vi "Teleop.vi"(10 "Match Info":T1={"Autonomous Elapsed Seconds"=0.0, "TeleOp Elapsed Seconds"=0.0, "Disabled Elapsed Seconds"=0.0, "Visited Autonomous"=FALSE, "Visited TeleOp"=FALSE, "Visited Disabled"=FALSE, "Autonomous Settings"={"Autonomous Style"=enum."Independent", "VI Refnum"=refnum}}, 11 "Call Context":T2) -> ()   [LabVIEW 2017]
doc: "This VI is called for each enabled TeleOp packet received from the DS. It is typically used to read from joysticks and other inputs and update I/O or setpoints for timed control loops. It should complete and return within 20 milliseconds or risk missing DS packets."
uses:
  <vilib>/Rock Robotics/WPI/DriverStation/WPI_DriverStationDerivedRobotMode.ctl
  <vilib>/Rock Robotics/WPI/DriverStation/WPI_DriverStationMatch Info.ctl
  <vilib>/Rock Robotics/WPI/Utilities/WPI_GetSetVariantRefNum.vi
  <vilib>/Rock Robotics/Network Tables/NT Write Boolean Array.vi
  <vilib>/Rock Robotics/Network Tables/NT Write Numeric Array.vi
  Framework/Robot Global Data.vi
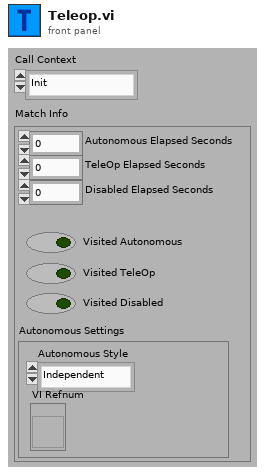
[diagram p1: front panel]
types:
  T1 = typedef "WPI_DriverStationMatch Info.ctl" = cluster{"Autonomous Elapsed Seconds":dbl, "TeleOp Elapsed Seconds":dbl, "Disabled Elapsed Seconds":dbl, "Visited Autonomous":bool, "Visited TeleOp":bool, "Visited Disabled":bool, "Autonomous Settings":cluster{"Autonomous Style":enum16{"Iterative", "Independent"}, "VI Refnum":refnum<vi>}}
  T2 = typedef "WPI_DriverStationDerivedRobotMode.ctl" = enum16{"Init", "Execute", "Stop"}
  T3 = typedef "WPI_JoystickDevRef.ctl" = cluster{"Device":T4}
  T4 = typedef "WPI_JoystickDeviceEnum.ctl" = enum16{"USB 0", "USB 1", "USB 2", "USB 3", "USB 4", "USB 5"}
  T5 = typedef "Command Status Info.ctl" = cluster{"Name":string, "Status":T6, "notifier out":T7}
  T6 = typedef "Completion Status.ctl" = enum16{"Successful", "Aborted", "Incomplete"}
  T7 = typedef "Completion Notifier.ctl" = refnum<notifier>
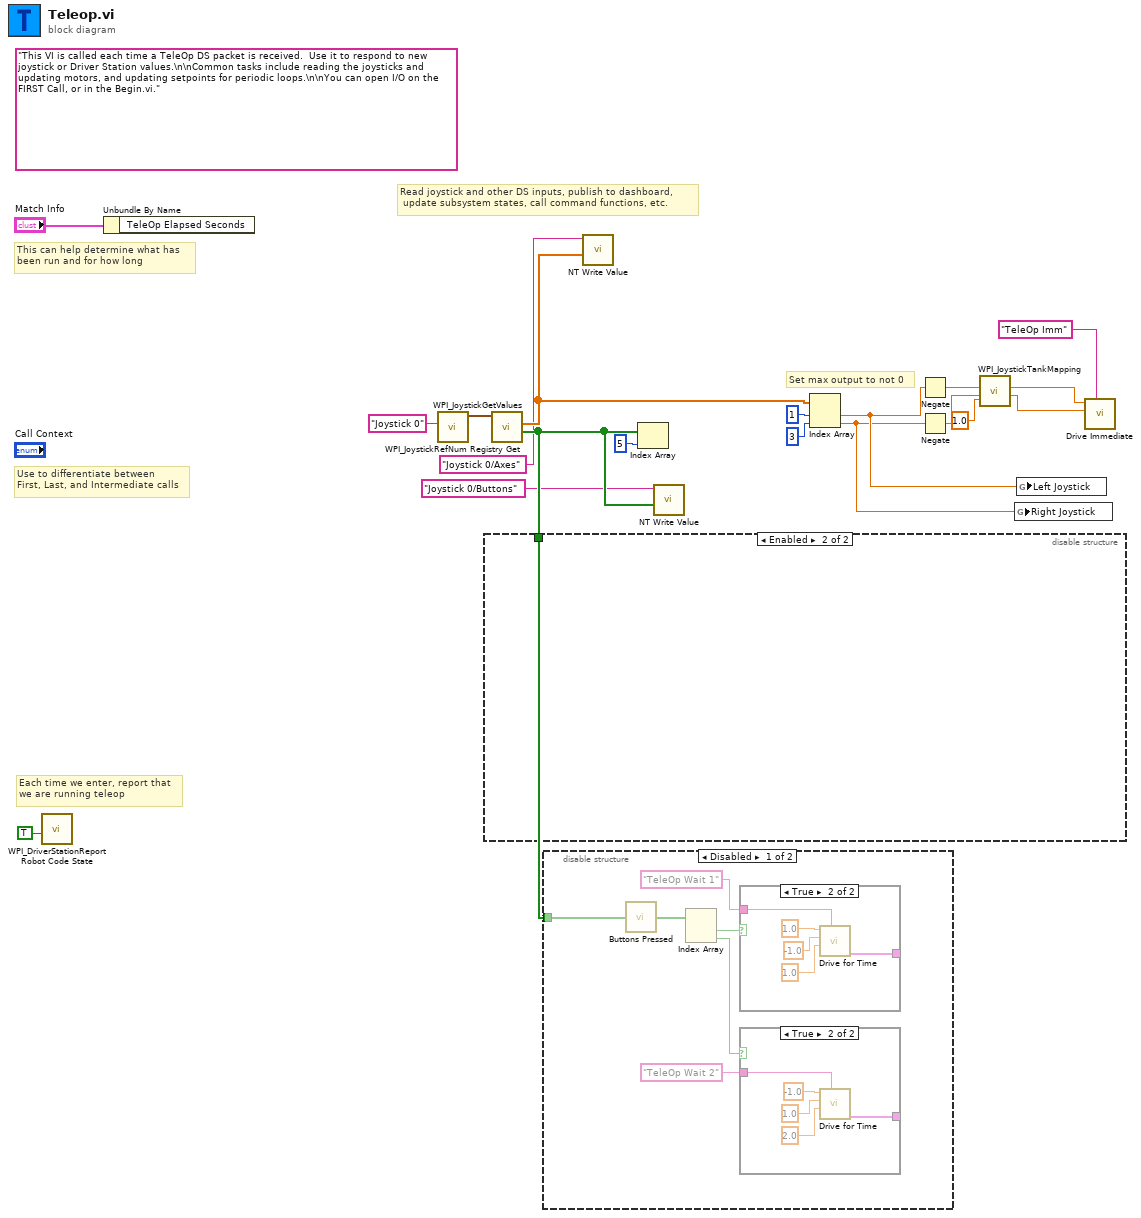
[diagram p0: block diagram]
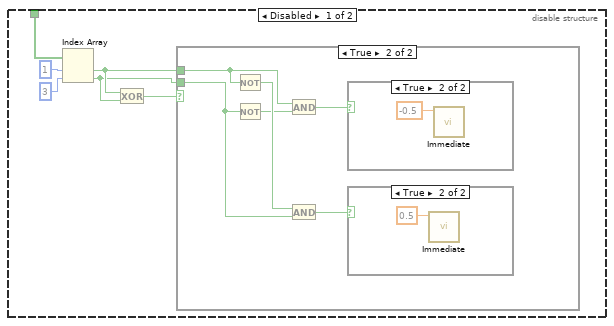
[diagram p2: hidden frame]
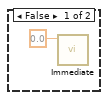
[diagram p3: hidden frame]
diagram:
  (unwired) "This VI is called each time a TeleOp DS packet is received.  Use it to respond to new joystick or Driver Station values.\n\nCommon tasks include reading the joysticks and updating motors, and updating setpoints for periodic loops.\n\nYou can open I/O on the FIRST Call, or in the Begin.vi."
  # "Set max output to not 0"
  # "Read joystick and other DS inputs, publish to dashboard,\n update subsystem states, call command functions, etc."
  # "Each time we enter, report that\nwe are running teleop"
  # "Use to differentiate between\nFirst, Last, and Intermediate calls"
  # "This can help determine what has\nbeen run and for how long"
  n1 = call <vilib>:"WPI_DriverStationReport Robot Code State.vi"("TeleOp"=TRUE ("Autonomous")) -> ()  [unwired: 10 in, 1 out]
  n2 = Unbundle By Name("Match Info") -> ()  [unwired: 1 out]
  n3 = call <vilib>:"WPI_JoystickRefNum Registry Get.vi"("refnum name"="Joystick 0") -> ("JoystickDevRef"=w16:T3)  [unwired: 1 in, 9 out]
  n4 = call <vilib>:"WPI_JoystickGetValues.vi"("JoystickDevRef"=w16) -> ("Buttons"=w15:bool[], "Axes"=w14:dbl[])  [unwired: 6 in, 3 out]
  n5 = disable-structure shown="Enabled" {
    disable-tunnel: w15 -> [w25 _]
    frame Disabled {
      n6 = Index Array(array=w25, index #1=1 ("index"), index #2=3 ("index")) -> (element #1=w24:bool, element #2=w23:bool)
      n7 = Exclusive Or(1:w23, 2:w24) -> (0:w20:bool)
      n8 = case shown="True" w20 {
        tunnel: w24 -> [_ w30]
        tunnel: w23 -> [_ w27]
        frame False {
          n9 = call "Immediate.vi"("Setpoint"=0.0) -> ()  [unwired: 10 in, 1 out]
        }
        frame True {
          n10 = Not(x=w30) -> (.not. x?=w31:bool)
          n11 = Not(x=w27) -> (.not. x?=w28:bool)
          n12 = And(x=w30, y=w28) -> (x .and. y?=w29:bool)
          n13 = And(x=w31, y=w27) -> (x .and. y?=w32:bool)
          n14 = case shown="True" w29 {
            frame False {
            }
            frame True {
              n15 = call "Immediate.vi"("Setpoint"=-0.5) -> ()  [unwired: 10 in, 1 out]
            }
          }
          n16 = case shown="True" w32 {
            frame False {
            }
            frame True {
              n17 = call "Immediate.vi"("Setpoint"=0.5) -> ()  [unwired: 10 in, 1 out]
            }
          }
        }
      }
    }
    frame Enabled {
    }
  }
  n18 = disable-structure shown="Disabled" {
    disable-tunnel: w15 -> [w35 _]
    frame Disabled {
      n19 = call "Buttons Pressed.vi"("Button Values"=w35) -> ("Button Presses"=w36:bool[])
      n20 = Index Array(array=w36) -> (element #1=w38:bool, element #2=w37:bool)  [unwired: 2 in]
      n21 = case shown="True" w38 {
        tunnel: [_ w49] -> _
        tunnel: "TeleOp Wait 1" ("Description") -> [_ w48]
        frame False {
        }
        frame True {
          n22 = call "Drive for Time.vi"("Description"=w48, "Seconds"=1.0, "Right Speed"=-1.0, "Left Speed"=1.0) -> ("Command Info Out"=w49:T5)  [unwired: 6 in, 1 out]
        }
      }
      n23 = case shown="True" w37 {
        tunnel: [_ w43] -> _
        tunnel: "TeleOp Wait 2" ("Description") -> [_ w42]
        frame False {
        }
        frame True {
          n24 = call "Drive for Time.vi"("Description"=w42, "Seconds"=2.0, "Right Speed"=1.0, "Left Speed"=-1.0) -> ("Command Info Out"=w43:T5)  [unwired: 6 in, 1 out]
        }
      }
    }
    frame Enabled {
    }
  }
  n25 = call-poly <vilib>:"NT Write Value.vi"("Numeric Array"=w14, "Name"="Joystick 0/Axes") -> ()  [unwired: 9 in, 1 out]
  n26 = Index Array(array=w15, index=5) -> ()  [unwired: 1 out]
  n27 = call-poly <vilib>:"NT Write Value.vi"("Boolean Array"=w15, "Name"="Joystick 0/Buttons") -> ()  [unwired: 9 in, 1 out]
  n28 = Index Array(array=w14, index #1=1 ("index"), index #2=3 ("index")) -> (element #1=w2:dbl, element #2=w1:dbl)
  n29 = Negate(x=w2) -> (-x=w4:dbl)
  n30 = Negate(x=w1) -> (-x=w3:dbl)
  n31 = call <vilib>:"WPI_JoystickTankMapping.vi"("Max Output"=1.0, "Right axis value"=w3, "Left axis value"=w4) -> ("Right Motor Value"=w9:dbl, "Left Motor Value"=w10:dbl)  [unwired: 7 in]
  n32 = global write "Robot Global Data.vi" "Right Joystick"(w1) -> ()
  n33 = global write "Robot Global Data.vi" "Left Joystick"(w2) -> ()
  n34 = call "Drive Immediate.vi"("Description"="TeleOp Imm", "Right Setpoint"=w9, "Left Setpoint"=w10) -> ()  [unwired: 8 in, 1 out]
